vi "Render.vi"(8 "error in (no error)":errorcluster, 11 "XRay Part Sample in":refnum<class "XRay Part Sample.lvclass">=refnum) -> (0 "error out":errorcluster, 2 "Scene Object":refnum<vi>, 3 "XRay Part Sample out":refnum<class "XRay Part Sample.lvclass">)   [LabVIEW 2026, in "XRay Part Sample.lvclass"]
uses:
  XRay Part Sample.lvclass
  XRay Table/XRay Table.lvclass
  XRay Part Sample.lvclass/XRay Part Sample.ctl
  <vilib>/picture/3D Picture Control/Object/Add Object (no reference).vi
  3D utilities/3D utilities.lvlib
  <vilib>/picture/3D Picture Control/NI_3D Picture Control.lvlib
panel:
  out "Mesh Size":i32=9438
  in  "Euler Angles":cluster{"phi":dbl, "theta":dbl, "psi":dbl}={"phi"=0.0, "theta"=180.0, "psi"=1.0} {"psi" scale=1.0..359.0; "theta" scale=0.0..360.0; "phi" scale=0.0..360.0}
  in  "scale":sgl=2.0
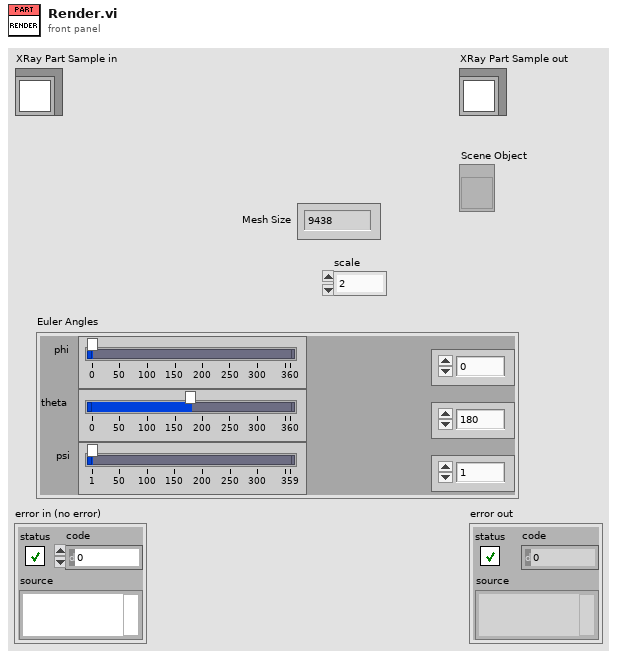
[diagram p1: front panel]
types:
  T1 = typedef "3DS Models.ctl" = enum16{"ASTM E2597 Step Wedge", "NI Bottle", "Utah Teapot", "Utah Teapot (Low Res)", "My Cube", "Tree", "Tree 2", "FreeCAD Sample", "Schenkel", "Bunny", "Corona Virus", "Corona Virus (Low Res)", "Offset"}
  T2 = enum16{"Inherit Value", "Points", "Wireframe", "Polygons"}
  T3 = typedef "NI_3D Picture Control.lvlib/NI_Old 3D Toolkit.lvlib/model.ctl" = cluster{"VertexList":T4[], "FaceList":cluster{"v1":i32, "v2":i32, "v3":i32}[], "NormalList":T4[], "Mode":T5}
  T4 = typedef "NI_3D Picture Control.lvlib/NI_Old 3D Toolkit.lvlib/point3f.ctl" = cluster{"x":sgl, "y":sgl, "z":sgl}
  T5 = typedef "NI_3D Picture Control.lvlib/NI_Old 3D Toolkit.lvlib/VertexMode.ctl" = enum16{"GL_POINTS", "GL_LINES", "GL_LINE_LOOP", "GL_LINE_STRIP", "GL_TRIANGLES", "GL_TRIANGLE_STRIP", "GL_TRIANGLE_FAN", "GL_QUADS", "GL_QUAD_STRIP", "GL_POLYGON"}
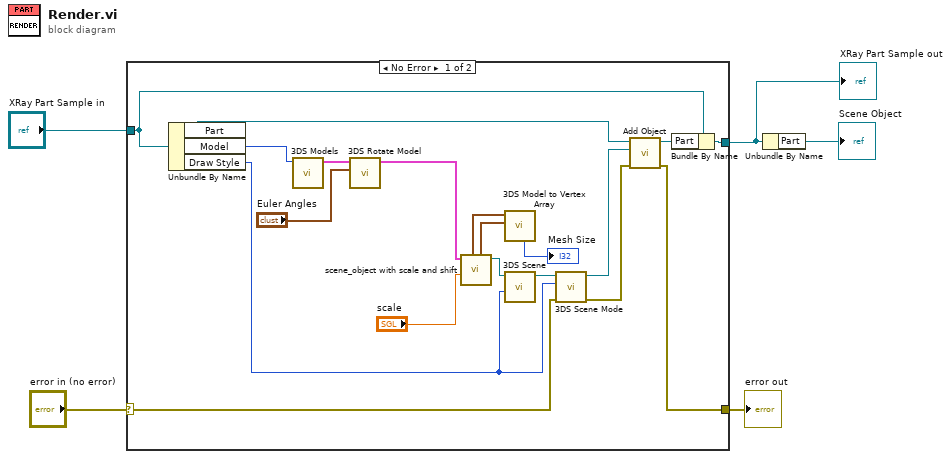
[diagram p0: block diagram]
diagram:
  n1 = case shown="No Error" "error in (no error)" {
    selector: "error in (no error)" -> [w8 w26]
    tunnel: [w6 w26] -> w4
    tunnel: [w14 w25] -> w2
    tunnel: "XRay Part Sample in" -> [w15 w25]
    frame No Error {
      n2 = Unbundle By Name(w15) -> ("Part"=w16:refnum<vi>, "Model"=w10:T1, "Draw Style"=w9:T2)
      n3 = call "3DS Models.vi"("Model"=w10) -> ("Model Out"=w20:T3)  [unwired: 10 in]
      n4 = call "3DS Rotate Model.vi"("Euler Angles"="Euler Angles", "model in"=w20) -> ("model out"=w21:T3)  [unwired: 9 in]
      n5 = call "scene_object with scale and shift.vi"("scale"="scale", "Object In"=w21) -> ("SceneMesh out"=w24:refnum<vi>, "FaceList"=w19:cluster{"v1":i32, "v2":i32, "v3":i32}[], "Array"=w18:T4[])  [unwired: 5 in, 2 out]
      n6 = call "3DS Model to Vertex Array.vi"("FaceList"=w19, "Array"=w18) -> ("Count"=→"Mesh Size":i32)  [unwired: 6 in, 3 out]
      n7 = call "3DS Scene.vi"("Draw Style:Mode"=w9, "SceneMesh in"=w24) -> ("SceneObject out"=w13:refnum<vi>)  [unwired: 8 in, 1 out]
      n8 = call "3DS Scene Mode.vi"("error in (no error)"=w8, "Draw Style:Mode"=w9, "SceneObject in"=w13) -> ("error out"=w7:errorcluster, "SceneObject out"=w12:refnum<vi>)  [unwired: 7 in]
      n9 = call-poly <vilib>:"Add Object.vi"("error in (no error)"=w7, "New Object In"=w12, "Scene Object In"=w16) -> ("error out"=w6:errorcluster, "Scene Object Out"=w11:refnum<vi>)  [unwired: 7 in]
      n10 = Bundle By Name(cluster=w15, "Part"=w11) -> (w14:refnum<class "XRay Part Sample.lvclass">)
    }
    frame Error {
    }
  }
  "error out" <- w4
  "XRay Part Sample out" <- w2
  n11 = Unbundle By Name(w2) -> ("Part"=→"Scene Object":refnum<vi>)
